vi "CREATE USER SQL QUERY.vi"(0 "What to Search":string, 5 "Search Column Name":string, 7 "Sorting Column Name":string, 9 "Column to Search In":u16, 12 "Date Range":u16(ring) items=["Greater Than", "Less Than", "Between"], 13 "Dates Less Than":string="8/1/2023", 14 "Dates Greater Than":string="8/1/2023") -> (4 "SQL QUERY":string)   [LabVIEW 2019]
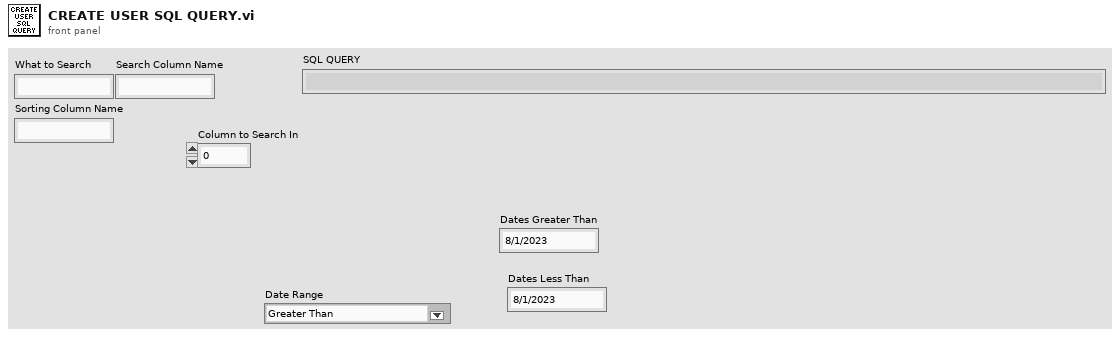
[diagram p1: front panel]
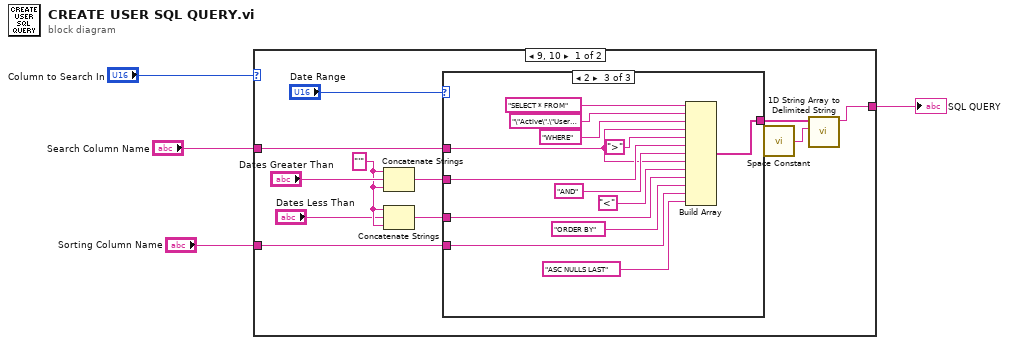
[diagram p0: block diagram]
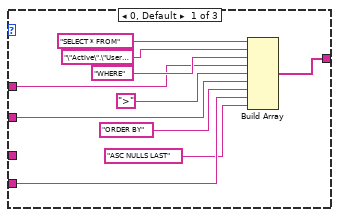
[diagram p2: hidden frame]
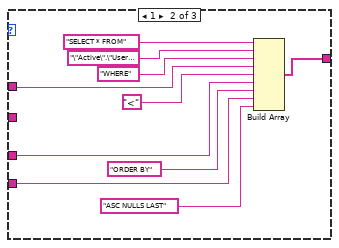
[diagram p3: hidden frame]
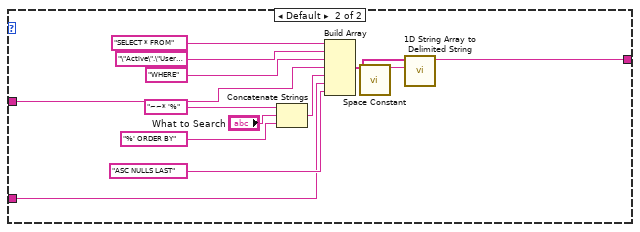
[diagram p4: hidden frame]
diagram:
  n1 = case shown="9, 10" "Column to Search In" {
    tunnel: "Search Column Name" -> [w14 w52]
    tunnel: "Sorting Column Name" -> [w10 w51]
    tunnel: [w13 w49] -> w1
    frame 9, 10 {
      w6 = "'"
      n2 = Concatenate Strings(w6, "Dates Greater Than", w6) -> (w9:string)
      n3 = Concatenate Strings(w6, "Dates Less Than", w6) -> (w8:string)
      n4 = case shown="2" "Date Range" {
        tunnel: w14 -> [w22 w29 w42]
        tunnel: w9 -> [w20 _ w44]
        tunnel: [w19 w26 w36] -> w12
        tunnel: w10 -> [w17 w28 w38]
        tunnel: w8 -> [_ w27 w40]
        frame 0, Default {
          n5 = Build Array("SELECT * FROM", "\"Active\".\"Users\"" ("string"), "WHERE" ("string"), w22, ">" ("string"), w20, "ORDER BY" ("string"), w17, "ASC NULLS LAST" ("string")) -> (w19:string[])
        }
        frame 1 {
          n6 = Build Array("SELECT * FROM", "\"Active\".\"Users\"" ("string"), "WHERE" ("string"), w29, "<" ("string"), w27, "ORDER BY" ("string"), w28, "ASC NULLS LAST" ("string")) -> (w26:string[])
        }
        frame 2 {
          n7 = Build Array("SELECT * FROM", "\"Active\".\"Users\"" ("string"), "WHERE" ("string"), w42, ">" ("string"), w44, "AND" ("string"), w42, "<" ("string"), w40, "ORDER BY" ("string"), w38, "ASC NULLS LAST" ("string")) -> (w36:string[])
        }
      }
      n8 = call <vilib>:"Space Constant.vi"() -> ("String"=w11:string)
      n9 = call <vilib>:"1D String Array to Delimited String.vi"("delimiter"=w11, "string array"=w12) -> ("delimited string"=w13:string)  [unwired: 9 in]
    }
    frame Default {
      n10 = Concatenate Strings("~~* '%" ("string"), "What to Search", "%' ORDER BY" ("string")) -> (w53:string)
      n11 = Build Array("SELECT * FROM", "\"Active\".\"Users\"" ("string"), "WHERE" ("string"), w52, w53, w51, "ASC NULLS LAST" ("string")) -> (w57:string[])
      n12 = call <vilib>:"Space Constant.vi"() -> ("String"=w50:string)
      n13 = call <vilib>:"1D String Array to Delimited String.vi"("delimiter"=w50, "string array"=w57) -> ("delimited string"=w49:string)  [unwired: 9 in]
    }
  }
  "SQL QUERY" <- w1
